vi "test1.vi"() -> ()   [LabVIEW 2017]
uses:
  MM-MotionSelect-CTRL.ctl
  <vilib>/picture/3D Picture Control/Object/Create Object (drawable).vi
  <vilib>/picture/3D Picture Control/Object/Add Object (reference).vi
  <vilib>/picture/3D Picture Control/NI_3D Picture Control.lvlib
panel:
  in  "startcapture":bool
  out "3D Picture":refnum<vi>(3d-picture)
  out "MotionChart":dbl[][](graph)
  in  "Motion.Select":T1
  in  "endprogram":bool
  in  "Set Analog Frequency":dbl=1500.0
  out "MotionBuffer":dbl[][][](array[numeric])
  out "Euler":dbl[][][](array[numeric])
  out "hardwaresetup?":bool
  in  "stopcapture":bool
  out "3DRef":refnum<vi>
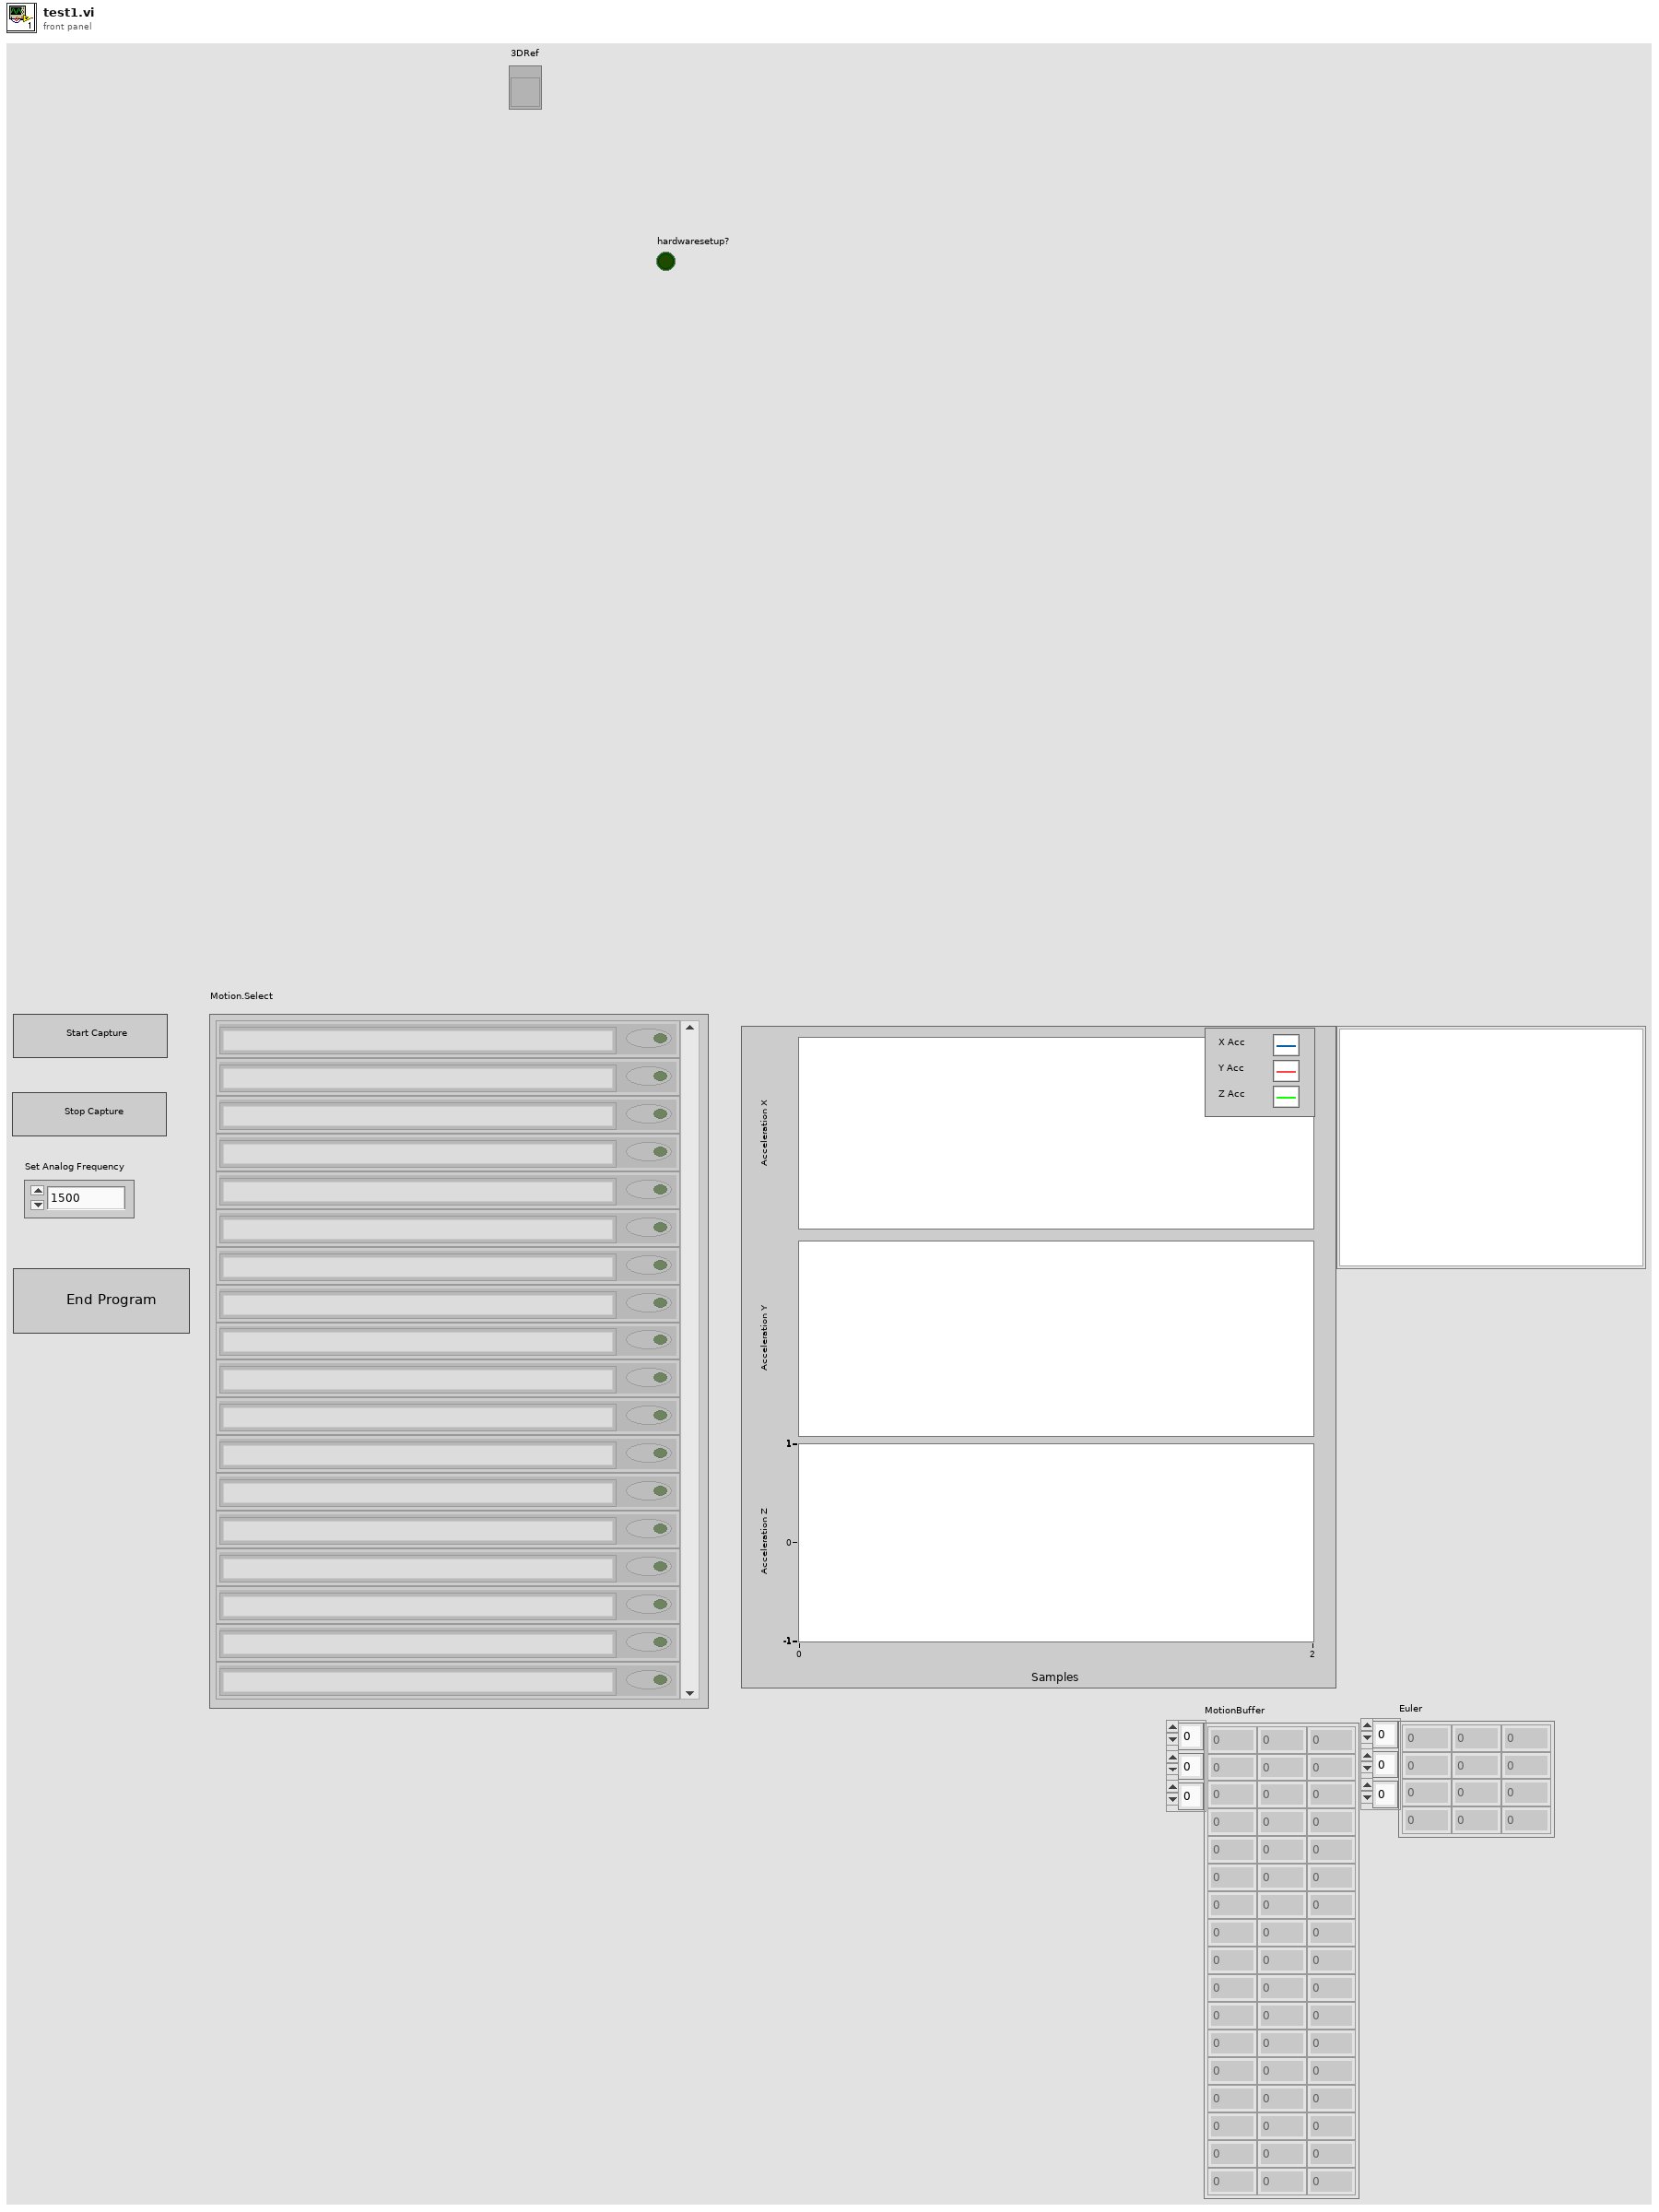
[diagram p1: front panel]
types:
  T1 = typedef "MM-MotionSelect-CTRL.ctl" = cluster{"Component":string, "Collect":bool}[]
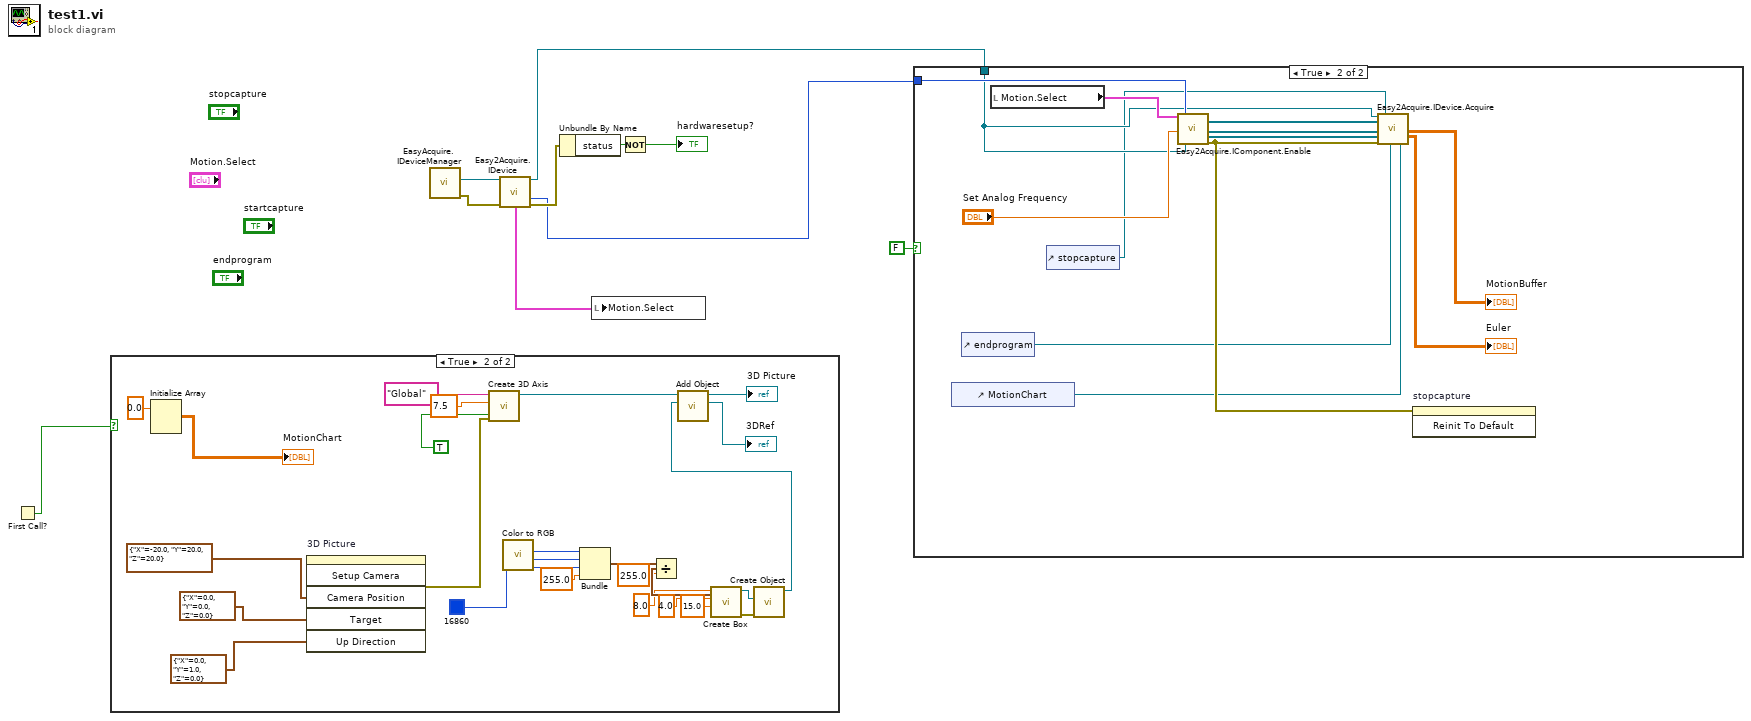
[diagram p0: block diagram]
diagram:
  n1 = First Call?() -> (First Call?: T/F=w10:bool)
  n2 = case shown="True" w10 {
    frame False {
    }
    frame True {
      n3 = Initialize Array(0.0 ("element")) -> (→"MotionChart":dbl[][])  [unwired: 2 in]
      n4 = invoke on="3D Picture" class="SceneGraphDisp (strict)" method="Setup Camera"("Camera Position"=cluster{"X":sgl, "Y":sgl, "Z":sgl} {"X"=-20.0, "Y"=20.0, "Z"=20.0}, "Target"=cluster{"X":sgl, "Y":sgl, "Z":sgl} {"X"=0.0, "Y"=0.0, "Z"=0.0}, "Up Direction"=cluster{"X":sgl, "Y":sgl, "Z":sgl} {"X"=0.0, "Y"=1.0, "Z"=0.0}) -> (error out=w16:errorcluster)  [unwired: 3 in, 5 out]
      n5 = call <vilib>:"Create 3D Axis.vi"("Axis label?"=TRUE, "error in (no error)"=w16, "Length"=sgl 7.5 ("Character Size"), "Name"="Global") -> ("New Object Refnum"=w20:refnum<vi>)  [unwired: 6 in, 1 out]
      n6 = call <vilib>:"Color to RGB.vi"("Color"=u32 16860 ("Color Box")) -> ("R"=w26:u8, "G"=w27:u8, "B"=w28:u8)  [unwired: 1 out]
      n7 = Bundle("R"=w26, "G"=w27, "B"=w28, 255.0) -> (w30:cluster{"R":u8, "G":u8, "B":u8, dbl})  [unwired: 1 in]
      n8 = Divide(x=w30, y=255.0) -> (x/y=w32:cluster{"R":dbl, "G":dbl, "B":dbl, dbl})
      n9 = call <vilib>:"Create Box.vi"("Color"=w32, "Length Z"=sgl 15.0, "Length Y"=sgl 4.0 ("Radius"), "Length X"=sgl 8.0 ("Height")) -> ("error out"=w23:errorcluster, "New Box Refnum"=w22:refnum<vi>)  [unwired: 6 in]
      n10 = call-poly <vilib>:"Create Object.vi"("error in (no error)"=w23, "Geometry"=w22) -> ("Scene:New Object"=w19:refnum<vi>)  [unwired: 8 in, 1 out]
      n11 = call-poly <vilib>:"Add Object.vi"("New Object In"=w19, "Scene Object In"=w20) -> ("New Object Out"=→"3DRef":refnum<vi>, "Scene Object Out"=→"3D Picture":refnum<vi>)  [unwired: 7 in, 1 out]
    }
  }
  n12 = call "EasyAcquire.IDeviceManager.vi"() -> ("error out"=w7:errorcluster, "GetCurrentDevice"=w9:refnum<k7>)  [unwired: 8 in, 2 out]
  n13 = call "Easy2Acquire.IDevice.vi"("IDeviceIn"=w9, "error in"=w7) -> ("IDeviceOut"=w3:refnum<k7>, "GetComponentCount"=w2:i32, "Motion.Select"=w8:T1, "error out"=w6:errorcluster)  [unwired: 8 in, 2 out]
  n14 = Unbundle By Name(w6) -> ("status"=w5:bool)
  n15 = local write "Motion.Select"(w8) -> ()
  n16 = Not(x=w5) -> (.not. x?=→"hardwaresetup?":bool)
  n17 = case shown="True" FALSE {
    tunnel: w2 -> [_ w48]
    tunnel: w3 -> [_ w46]
    frame False {
    }
    frame True {
      n18 = control-ref of="MotionChart"() -> (w41:refnum<vi>)
      n19 = control-ref of="endprogram"() -> (w40:refnum<vi>)
      n20 = local read "Motion.Select"() -> (w49:T1)
      n21 = control-ref of="stopcapture"() -> (w39:refnum<vi>)
      n22 = call "Easy2Acquire.IComponent.Enable.vi"("Motion.Select"=w49, "AnalogFreq"="Set Analog Frequency", "ComponentCount"=w48, "IDeviceIn"=w46) -> ("AnalogInput"=w45:refnum<k7>[], "DigitalInput"=w44:refnum<k7>[], "MotionInput"=w43:refnum<k7>[], "error out"=w42:errorcluster)  [unwired: 12 in]
      n23 = call "Easy2Acquire.IDevice.Acquire.vi"("IDeviceIn"=w46, "IAnalogInput"=w45, "DigitalInput"=w44, "MotionInput"=w43, "error in (no error)"=w42, "stopcapture"=w39, "endprogram"=w40, "MotionChart"=w41) -> ("MotionBuffer"=→"MotionBuffer":dbl[][][], "Euler"=→"Euler":dbl[][][])  [unwired: 8 in, 2 out]
      n24 = invoke on="stopcapture" class="Bool (strict)" method="Reinit To Default"(error in=w42) -> ()  [unwired: 2 in, 3 out]
    }
  }
